vi "UHR-Fleezers Control (host) -Leonardo 04-2018 V3.vi"(0 "Tab Control":T5(tab)=enum."Trap Control (RF)") -> ()   [LabVIEW 2013] (continued)
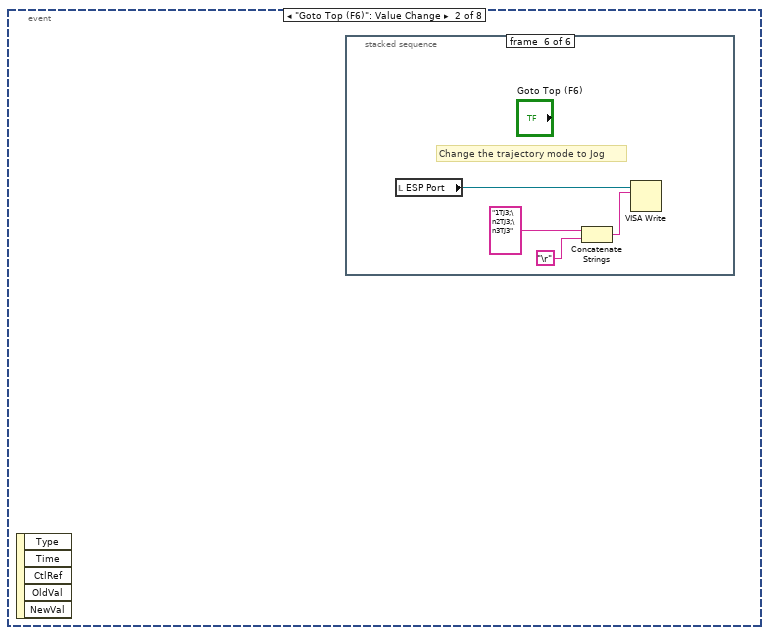
[diagram p4: hidden frame]
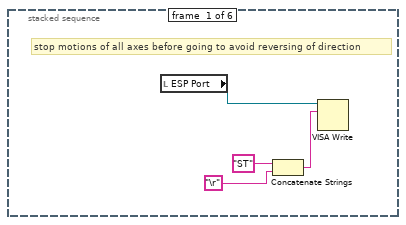
[diagram p5: hidden frame]
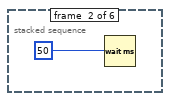
[diagram p6: hidden frame]
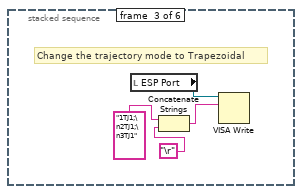
[diagram p7: hidden frame]
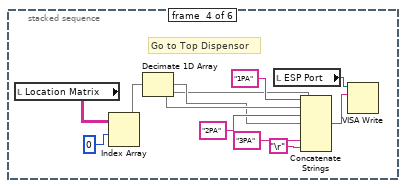
[diagram p8: hidden frame]
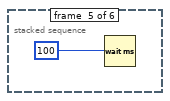
[diagram p9: hidden frame]
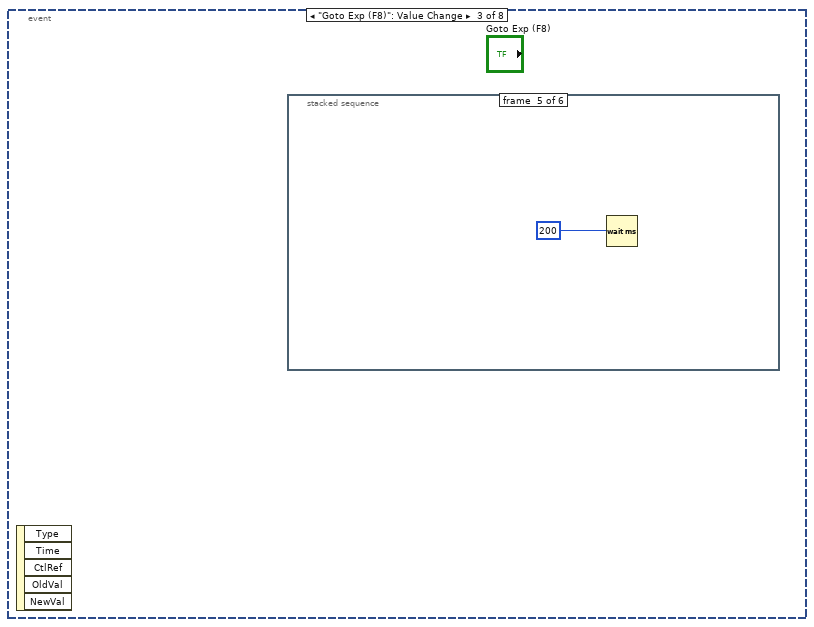
[diagram p10: hidden frame]
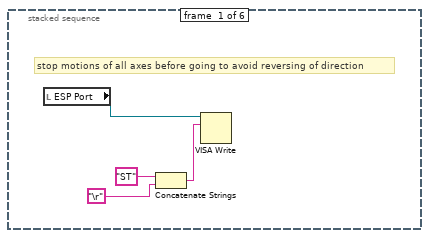
[diagram p11: hidden frame]
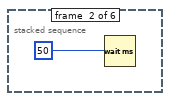
[diagram p12: hidden frame]
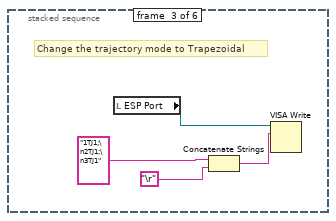
[diagram p13: hidden frame]
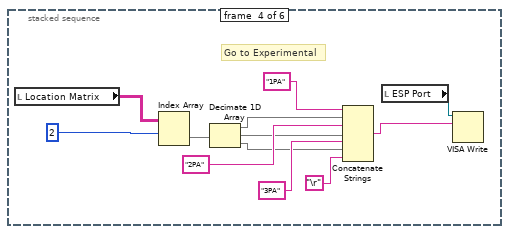
[diagram p14: hidden frame]
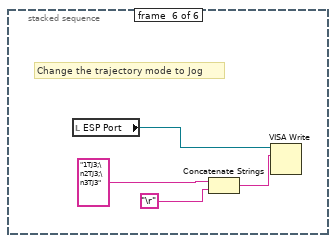
[diagram p15: hidden frame]
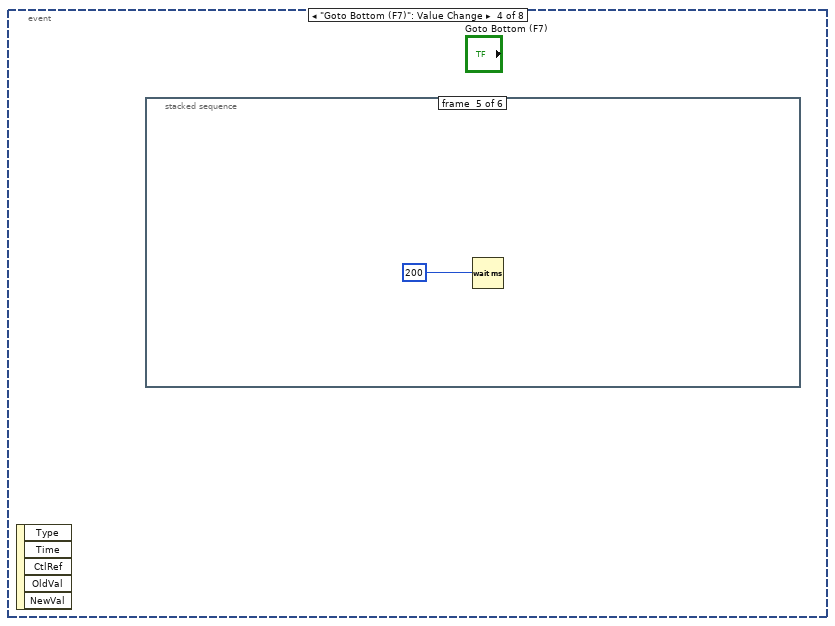
[diagram p16: hidden frame]
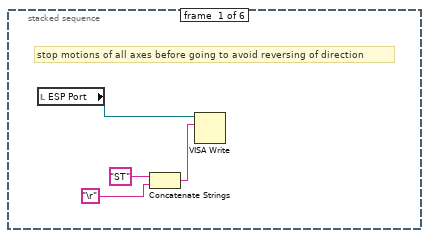
[diagram p17: hidden frame]
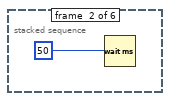
[diagram p18: hidden frame]
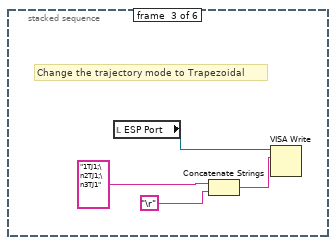
[diagram p19: hidden frame]
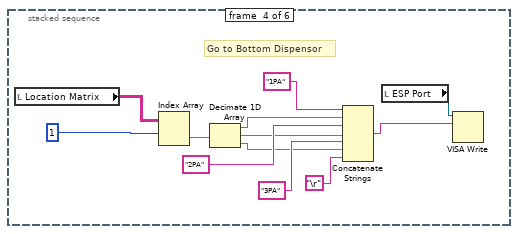
[diagram p20: hidden frame]
                n2319 = Write to Binary File(file (use dialog)=w3910, data=w3903, 5:FALSE ("prepend array or string size? (T)"), 9:T30."big-endian, network order" ("byte order (0:big-endian, network order)")) -> ()  [unwired: 1 in, 4 out]
                n2320 = feedback #26(w3876) -> (w3878:dbl[])
                n2321 = Build Array (concatenate)(w3878, w3876) -> (w3877:dbl[])
                n2322 = Select(t=w3876, s=w3852, f=w3877) -> (s? t:f=w3862:dbl[])
                n2323 = feedback-in #26(w3862) -> ()
                n2324 = feedback #27(w3884) -> (w3897:dbl[])
                n2325 = Build Array (concatenate)(w3897, w3884) -> (w3896:dbl[])
                n2326 = Select(t=w3884, s=w3852, f=w3896) -> (s? t:f=w3871:dbl[])
                n2327 = feedback-in #27(w3871) -> ()
                n2328 = Divide(x=w3911, y=w3912) -> (x/y=w3914:dbl)
                n2329 = Multiply(x=w3914, y=100.0) -> (x*y=w3913:dbl)
                n2330 = Build Array(w3871, w3862) -> (→"Saved APD":dbl[][])
                n2331 = Array Size(array=w3871) -> (size(s)=w3889:i32)
                n2332 = Unbundle By Name(w3891) -> ("Y"=w3895:dbl[])
                n2333 = Subtract(x=w3889, y="N pts to average") -> (x-y=w3865:i32)
                n2334 = Multiply(x="N pts to average", y=u16 2) -> (x*y=w3866:u16)
                n2335 = Subtract(x=w3889, y=w3866) -> (x-y=w3864:i32)
                n2336 = feedback #28(w3895) -> (w3894:dbl[])
                n2337 = Build Array (concatenate)(w3894, w3895) -> (w3893:dbl[])
                n2338 = Select(t=w3895, s=w3852, f=w3893) -> (s? t:f=w3892:dbl[])
                "Trap Delta Graph" <- w3892
                n2339 = feedback-in #28(w3892) -> ()
                n2340 = Array Subset(array=w3871, index=w3865, length="N pts to average") -> (w3888:dbl[])
                n2341 = Array Subset(array=w3871, index=w3864, length="N pts to average") -> (w3887:dbl[])
                n2342 = Array Subset(array=w3862, index=w3865, length="N pts to average") -> (w3868:dbl[])
                n2343 = Array Subset(array=w3862, index=w3864, length="N pts to average") -> (w3867:dbl[])
                n2344 = call-poly <vilib>:"Mean.vi"("X"=w3888) -> ("mean"=w3886:dbl)  [unwired: 1 out]
                n2345 = call-poly <vilib>:"Mean.vi"("X"=w3868) -> ("mean"=w3861:dbl)  [unwired: 1 out]
                n2346 = call-poly <vilib>:"Mean.vi"("X"=w3887) -> ("mean"=w3885:dbl)  [unwired: 1 out]
                n2347 = call-poly <vilib>:"Mean.vi"("X"=w3867) -> ("mean"=w3860:dbl)  [unwired: 1 out]
                n2348 = Subtract(x=w3861, y=w3860) -> (x-y=w3851:dbl)
                "Delta Fl. 2" <- w3851
                n2349 = Subtract(x=w3886, y=w3885) -> (x-y=w3883:dbl)
                "Delta Fl. 1" <- w3883
                n2350 = Initialize Array(w3883, 1 ("dimension size")) -> (w3880:dbl[])
                n2351 = Initialize Array(w3851, 1 ("dimension size")) -> (w3857:dbl[])
                n2352 = feedback #29(w3880) -> (w3881:dbl[])
                n2353 = Build Array (concatenate)(w3881, w3880) -> (w3879:dbl[])
                n2354 = feedback #30(w3857) -> (w3858:dbl[])
                n2355 = Build Array (concatenate)(w3858, w3857) -> (w3856:dbl[])
                n2356 = Select(t=w3880, s=w3852, f=w3879) -> (s? t:f=w3855:dbl[])
                n2357 = feedback-in #29(w3855) -> ()
                n2358 = Select(t=w3857, s=w3852, f=w3856) -> (s? t:f=w3854:dbl[])
                n2359 = feedback-in #30(w3854) -> ()
                n2360 = Build Array(w3855, w3854) -> (→"Save APD Deriv":dbl[][])
              }
            }
            "Progress" <- w3828
            "Progress 2" <- w3828
          }
        }
      }
    }
    n2361 = Divide(x=w2209, y=w2210) -> (x/y=w2200:ext)
    "Trap 2 amplitude" <- w2200
    n2362 = Bundle By Name(cluster=w2463, "Green FB Ch 0"=w2462, "Green FB Ch 1"=w2461) -> (w2447:T49)
    "Green FB Signals (V)" <- w2447
    n2363 = case shown="True" w2202 {
      tunnel: w2201 -> [_ w2552]
      tunnel: w2200 -> [_ w2551]
      frame False {
      }
      frame True {
        w2553 = 50.0
        n2364 = Greater?(x=w2551, y=w2553) -> (0:w2549:bool)
        n2365 = Greater?(x=w2552, y=w2553) -> (0:w2550:bool)
        n2366 = Or(x=w2550, y=w2549) -> (x .or. y?=w2548:bool)
        n2367 = case shown="True" w2548 {
          frame False {
          }
          frame True {
            n2368 = property on="All FB On/Off" class="Bool (strict)"("Val(Sgnl)"=FALSE) -> ()  [unwired: 2 in, 2 out]
            "Feedback overload" <- TRUE
          }
        }
      }
    }
    n2369 = Unbundle By Name(w2447) -> ("Green FB Ch 2"=→"Green FB Plot":dbl)
    n2370 = local read "wait to reset values"() -> (w2531:bool)
    n2371 = Not(x=w2528) -> (.not. x?=w2532:bool)
    n2372 = And(x=w2532, y=w2531) -> (x .and. y?=w2533:bool)
    n2373 = case "Part of MCL raster scanning: returns to initial positions after scan done" shown="True" w2533 {
      tunnel: w2536 -> [w3377 w3384]
      tunnel: [w3377 w3383] -> w2535
      tunnel: w2530 -> [w3376 w3382]
      tunnel: [w3376 w3381] -> w2529
      frame False {
      }
      frame True {
        w3392 = 10.0 ("y")
        w3391 = 32767.0 ("y")
        # "to return scan values\nafter a synchronous \nAOM scan"
        n2374 = local read "AO2"() -> (w3385:dbl)
        n2375 = local read "AO1"() -> (w3386:dbl)
        n2376 = local write "wait to reset values"(FALSE ("wait to reset values")) -> ()
        n2377 = Multiply(x=w3386, y=w3391) -> (x*y=w3388:dbl)
        n2378 = Multiply(x=w3385, y=w3391) -> (x*y=w3390:dbl)
        n2379 = Divide(x=w3388, y=w3392) -> (x/y=w3387:dbl)
        n2380 = Divide(x=w3390, y=w3392) -> (x/y=w3389:dbl)
        n2381 = To Word Integer(number=w3387) -> (16bit integer=w3393:i16)
        n2382 = To Word Integer(number=w3389) -> (16bit integer=w3394:i16)
        n2383 = local read "Total Counts (ticks)"() -> (w3378:u32)
        n2384 = xnode "Read/Write Control"("FPGA VI Reference In"=w3384, "error in"=w3382, "AO1 (Y)"=w3393, "AO2 (X)"=w3394, "MCL count"=w3378) -> ("FPGA VI Reference Out"=w3383:T20, "error out"=w3381:errorcluster)
        n2385 = local read "Scan Range (V)\n(of steps)"() -> (w3379:dbl)
        n2386 = property on="Scan Range (V)\n(of steps)" class="DigNum (strict)"("Val(Sgnl)"=w3379) -> ()  [unwired: 2 in, 2 out]
      }
    }
    n2387 = node-c288() -> ()  [unwired: 2 out]
  }
  n2388 = node-c288(3 ("Processor")) -> (w107:T25)  [unwired: 3 out]
  n2389 = timed-loop "Oscillate AOD (debugging)" {
    tunnel: w57 -> [w3956]
    tunnel: [w3955] -> w69
    timing: w107 -> [_]
    timing-out: [_] -> w106
    stop <- w3955 stop-if-true
    n2390 = node-c288() -> ()  [unwired: 2 out]
    n2391 = event shown="[0] \"Oscillate Set 2\", \"Fish for Tether\": Value Change" {
      selector: _ -> [_ _ _]
      dyn-events: _ -> [_ _ _]
      timeout: _ -> [_ _ _]
      tunnel: w3956 -> [w3963 _ _]
      tunnel: [FALSE ("Stop All") _ w4231] -> w3955
      event "Oscillate Set 2", "Fish for Tether": Value Change {
        n2392 = event-data() -> ()  [unwired: 6 out]
        n2393 = local read "Oscillate Set 2"() -> (w3962:bool)
        n2394 = Or(x=w3962, y="Fish for Tether") -> (x .or. y?=w3960:bool)
        n2395 = case shown="True" w3960 {
          tunnel: w3963 -> [_ w3966]
          tunnel: "Fish for Tether" -> [_ w3965]
          frame False {
          }
          frame True {
            n2396 = case shown="True" w3965 {
              frame False {
              }
              frame True {
                n2397 = local write "Scan axis 2"(TRUE) -> ()
                n2398 = local write "Tether"(FALSE ("Tether")) -> ()
              }
            }
            n2399 = node-c288("Period") -> (w3968:T25)  [unwired: 3 out]
            n2400 = timed-loop "Oscillate AOD" {
              timing: w3968 -> [_]
              timing-out: [_] -> w3967
              tunnel: w3966 -> [w3978]
              tunnel: w3965 -> [w3977]
              i -> [w3980]
              stop <- w3976 stop-if-true
              n2401 = node-c288() -> (w3979:i64)  [unwired: 1 out]
              n2402 = flat-sequence {
                tunnel: w3980 -> [w4006]
                tunnel: w3979 -> [w4005]
                tunnel: w3978 -> [w3989]
                tunnel: w3977 -> [w3991]
                tunnel: [w3991] -> w3975
                tunnel: [w3990] -> w3974
                tunnel: [w3988] -> w3973
                tunnel: [w3985] -> w3971
                tunnel: w3975 -> [w4042]
                tunnel: w3974 -> [w4040]
                tunnel: w3973 -> [w4039]
                tunnel: [w4038] -> w3972
                tunnel: w3971 -> [w4037]
                tunnel: [w4106] -> w3976
                tunnel: w3972 -> [w4104]
                frame #0 {
                  n2403 = Divide(x=w4005, y=i64 1000) -> (x/y=w4000:dbl)
                  n2404 = Multiply(x=w4000, y=w4006) -> (x*y=w4002:dbl)
                  n2405 = Multiply(x="Osc. freq. (Hz)", y=6.283185307179586) -> (x*y=w4003:dbl)
                  n2406 = Multiply(x=w4003, y=w4002) -> (x*y=w3987:dbl)
                  n2407 = local read "BD 1 Frequency 2 (MHz)"() -> (w3984:dbl)
                  n2408 = local read "BD 1 Frequency 1 (MHz)"() -> (w3981:dbl)
                  n2409 = case shown="True" w3991 {
                    tunnel: w3987 -> [w4012 w4019]
                    tunnel: w3984 -> [_ w4029]
                    tunnel: [w4009 w4013] -> w3992
                    tunnel: [FALSE w4022] -> w3988
                    tunnel: [0.0 w4015] -> w3985
                    tunnel: w3981 -> [_ w4014]
                    frame False {
                      n2410 = Sine(x=w4012) -> (sin(x)=w4010:dbl)
                      n2411 = Multiply(x=w4010, y="Osc. amp. (MHz)") -> (x*y=w4009:dbl)
                    }
                    frame True {
                      n2412 = Cosine(x=w4019) -> (cos(x)=w4032:dbl)
                      n2413 = Subtract(x=w4029, y=w4014) -> (x-y=w4028:dbl)
                      n2414 = Decrement(x=w4032) -> (x-1=w4031:dbl)
                      n2415 = Subtract(x=w4028, y="Closest Delta (MHz)") -> (x-y=w4025:dbl)
                      n2416 = Divide(x=w4031, y=2.0) -> (x/y=w4026:dbl)
                      n2417 = Multiply(x=w4026, y=w4025) -> (x*y=w4013:dbl)
                      n2418 = local read "Vec Mean of T1 T2"() -> (w4021:dbl[])
                      n2419 = Greater?(x=w4021, y="Stop F (pN)") -> (0:w4023:bool[])
                      n2420 = Or Array Elements(Boolean array=w4023) -> (logical OR=w4022:bool)
                      n2421 = Divide(x=w4019, y=6.283185307179586) -> (x/y=w4018:dbl)
                      n2422 = Round Toward +Infinity(x=w4018) -> (ceil(x): smallest int >= x=w4015:dbl)
                      "Attempts" <- w4015
                      n2423 = Greater?(x=w4015, y="Attempt Limit") -> (0:w4017:bool)
                      n2424 = case shown="True" w4017 {
                        frame False {
                        }
                        frame True {
                          n2425 = local write "Fish for Tether"(FALSE ("Fish for Tether")) -> ()
                          n2426 = call <vilib>:"Beep.vi"() -> ()  [unwired: 3 in, 9 out]
                          n2427 = local read "Messages"() -> (w4034:string)
                          n2428 = call "Update messages.vi"("Message to add"="Tether fishing timeout." ("Messages"), "Old message string"=w4034) -> ("New message string"=→"Messages":string)
                        }
                      }
                    }
                  }
                  n2429 = local read "Y RF Frequency Limits (MHz)"() -> (w3993:T16)
                  n2430 = local read "X RF Frequency Limits (MHz)"() -> (w3994:T16)
                  n2431 = local read "BD 1 Frequency 3 (MHz)"() -> (w3999:dbl)
                  n2432 = local read "BD 2 Frequency 2 (MHz)"() -> (w3983:dbl)
                  n2433 = Select(t=w3984, s="Scan axis 2", f=w3983) -> (s? t:f=w3995:dbl)
                  n2434 = Add(x=w3992, y=w3995) -> (x+y=w3990:dbl)
                  n2435 = Select(t=w3990, s="Scan axis 2", f=w3984) -> (s? t:f=w3982:dbl)
                  n2436 = Select(t=w3983, s="Scan axis 2", f=w3990) -> (s? t:f=w3997:dbl)
                  n2437 = local read "BD 2 Frequency 3 (MHz)"() -> (w3998:dbl)
                  n2438 = call "set RF board frequency - interlace.vi"("Board 2 Frequency Limits"=w3993, "Board 1 Frequency Limits"=w3994, "FPGA VI Reference In"=w3989, "Board 2 Frequency 3 (MHz)"=w3998, "Board 1 Frequency 3 (MHz)"=w3999, "Board 2 Frequency 2 (MHz)"=w3983, "Board 2 Frequency 1 (MHz)"=w3997, "Board 1 Frequency 2 (MHz)"=w3982, "Board 1 Frequency 1  (MHz)"=w3981) -> ()  [unwired: 1 in, 2 out]
                }
                frame #1 {
                  n2439 = And(x=w4042, y=w4039) -> (x .and. y?=w4041:bool)
                  n2440 = case "Only if were fishing and now formed tether" shown="True" w4041 {
                    tunnel: w4040 -> [w4044 w4056]
                    tunnel: [w4043 w4055] -> w4038
                    tunnel: w4037 -> [_ w4051]
                    frame False {
                      n2441 = local read "Fish for Tether"() -> (w4043:bool)
                      n2442 = case shown="True" w4043 {
                        tunnel: w4044 -> [_ _]
                        frame False {
                        }
                        frame True {
                        }
                      }
                    }
                    frame True {
                      w4055 = FALSE ("Fish for Tether")
                      n2443 = call <vilib>:"Beep.vi"() -> ()  [unwired: 3 in, 9 out]
                      n2444 = Number To Decimal String(number=w4051, width (-)=i16 1) -> (decimal integer string=w4049:string)
                      n2445 = case shown="\"2\", \"3\", \"4\", \"5\", \"6\"" "Then..." {
                        selector: "Then..." -> [_ w4059]
                        tunnel: w4056 -> [w4058 _]
                        frame "1", Default {
                          # "do nothing"
                          n2446 = property on="BD 1 Frequency 1 (MHz)" class="DigNum (strict)"("Val(Sgnl)"=w4058) -> ()  [unwired: 2 in, 2 out]
                        }
                        frame "2", "3", "4", "5", "6" {
                          n2447 = flat-sequence {
                            tunnel: w4059 -> [w4061]
                            frame #0 {
                              n2448 = property on="Trap Delta (MHz)" class="DigNum (strict)"("Val(Sgnl)"="Move to Delta 1 (MHz)") -> ()  [unwired: 2 in, 2 out]
                            }
                            frame #1 {
                              n2449 = case shown="\"5\", \"6\"" w4061 {
                                selector: w4061 -> [w4064 w4074 _]
                                frame "3", "4" {
                                n2450 = flat-sequence {
                                tunnel: w4064 -> [w4065]
                                tunnel: [w4065] -> w4062
                                tunnel: [w4067] -> w4063
                                tunnel: w4062 -> [w4067]
                                tunnel: w4063 -> [w4071]
                                frame #0 {
                                n2451 = property on="Green Laser ON/Interlacing" class="Bool (strict)"("Val(Sgnl)"=TRUE ("Value (Signaling)")) -> ()  [unwired: 2 in, 2 out]
                                }
                                frame #1 {
                                n2452 = Multiply(x="Wait Before Save (s)", y=u32 1000 ("x")) -> (x*y=w4069:u32)
                                n2453 = Wait (ms)(milliseconds to wait=w4069) -> ()  [unwired: 1 out]
                                }
                                frame #2 {
                                n2454 = property on="Start Saving" class="Bool (strict)"("Value"=TRUE ("Start Saving")) -> ()  [unwired: 2 in, 2 out]
                                n2455 = case shown="Default" w4071 {
                                frame Default {
                                }
                                frame "4" {
                                n2456 = property on="Fl. Triggered..." class="Bool (strict)"("Val(Sgnl)"=TRUE ("Value (Signaling)")) -> ()  [unwired: 2 in, 2 out]
                                }
                                }
                                }
                                }
                                }
                                frame "5", "6" {
                                n2457 = stacked-sequence {
                                tunnel: w4074 -> [_ _ _ _ _ _ _ _ w4091 _ _]
                                frame #0 {
                                n2458 = Replace Array Subset(array=u32[] [0] ("Index Values"), new element="Raster Set Upon Tether", index=0) -> (w4075:u32[])
                                n2459 = property on="Saved AOD Raster Scan Parameter Sets" class="Arr (strict)"("Index Values"=w4075) -> ()  [unwired: 2 in, 2 out]
                                }
                                frame #1 {
                                n2460 = Wait (ms)(milliseconds to wait=u32 500) -> ()  [unwired: 1 out]
                                }
                                frame #2 {
                                n2461 = property on="Load parameters" class="Bool (strict)"("Val(Sgnl)"=TRUE ("Value (Signaling)")) -> ()  [unwired: 2 in, 2 out]
                                }
                                frame #3 {
                                n2462 = Wait (ms)(milliseconds to wait=u32 500) -> ()  [unwired: 1 out]
                                }
                                frame #4 {
                                n2463 = property on="Trap Raster Scan" class="Bool (strict)"("Val(Sgnl)"=TRUE ("Value (Signaling)")) -> ()  [unwired: 2 in, 2 out]
                                }
                                frame #5 {
                                n2464 = Wait (ms)(milliseconds to wait=u32 2000) -> ()  [unwired: 1 out]
                                }
                                frame #6 {
                                n2465 = while {
                                stop <- w4086 stop-if-true
                                n2466 = local read "Raster Scanning..."() -> (w4085:bool)
                                n2467 = local read "Saving..."() -> (w4088:bool)
                                n2468 = Wait (ms)(milliseconds to wait=u32 100) -> ()  [unwired: 1 out]
                                n2469 = Not(x=w4088) -> (.not. x?=w4087:bool)
                                n2470 = Not(x=w4085) -> (.not. x?=w4084:bool)
                                n2471 = And(x=w4087, y=w4084) -> (x .and. y?=w4086:bool)
                                }
                                }
                                frame #7 {
                                n2472 = property on="Trap Delta (MHz)" class="DigNum (strict)"("Val(Sgnl)"="Move to Delta 2 (MHz)") -> ()  [unwired: 2 in, 2 out]
                                }
                                frame #8 {
                                n2473 = local read "Tether"() -> (w4092:bool)
                                n2474 = case shown="True" w4092 {
                                tunnel: w4091 -> [_ w4093]
                                frame False {
                                }
                                frame True {
                                n2475 = flat-sequence {
                                tunnel: w4093 -> [w4095]
                                frame #0 {
                                n2476 = Wait (ms)(milliseconds to wait=u32 500) -> ()  [unwired: 1 out]
                                }
                                frame #1 {
                                n2477 = case shown="\"6\"" w4095 {
                                frame Default {
                                }
                                frame "6" {
                                n2478 = property on="Green Laser ON/Interlacing" class="Bool (strict)"("Val(Sgnl)"=TRUE ("Green Laser ON/Interlacing")) -> ()  [unwired: 2 in, 2 out]
                                }
                                }
                                }
                                frame #2 {
                                n2479 = Wait (ms)(milliseconds to wait=u32 500) -> ()  [unwired: 1 out]
                                }
                                frame #3 {
                                n2480 = local write "Start Saving"("Save at end (5, 6)") -> ()
                                }
                                }
                                }
                                }
                                }
                                frame #9 {
                                n2481 = local read "Bead Sep. Int. Time (s)"() -> (w4101:dbl)
                                n2482 = Multiply(x=w4101, y=1000.0) -> (x*y=w4100:dbl)
                                n2483 = Wait (ms)(milliseconds to wait=w4100) -> ()  [unwired: 1 out]
                                }
                                frame #10 {
                                n2484 = property on="Rescale on Mean" class="Bool (strict)"("Val(Sgnl)"=TRUE ("Value (Signaling)")) -> ()  [unwired: 2 in, 2 out]
                                }
                                }
                                }
                                frame "2", Default {
                                }
                              }
                            }
                          }
                        }
                      }
                      n2485 = Concatenate Strings("Formed tether in ", w4049, " attempt(s)." ("string")) -> (w4046:string)
                      n2486 = local read "Messages"() -> (w4053:string)
                      n2487 = local write "Fish for Tether"(w4055) -> ()
                      n2488 = call "Update messages.vi"("Message to add"=w4046, "Old message string"=w4053) -> ("New message string"=w4052:string)
                      n2489 = local write "Messages"(w4052) -> ()
                      n2490 = Get Date/Time In Seconds() -> (seconds since 1Jan1904=→"Time tether formed":timestamp)
                      "Tether" <- "Tether Alarm?"
                    }
                  }
                }
                frame #2 {
                  n2491 = local read "Oscillate Set 2"() -> (w4105:bool)
                  n2492 = local read "Stop All"() -> (w4107:bool)
                  n2493 = Not Or(1:w4104, 2:w4105) -> (0:w4103:bool)
                  n2494 = Compound Arithmetic op=OR(w4107, w4103) -> (w4106:bool)
                }
              }
              n2495 = node-c288() -> ()  [unwired: 2 out]
            }
            n2496 = node-c288(w3967) -> ()  [unwired: 1 out]
          }
        }
      }
      event "Fl. Triggered...": Value Change {
        n2497 = event-data() -> ()  [unwired: 7 out]
        n2498 = case shown="True" "Fl. Triggered..." {
          frame False {
          }
          frame True {
            n2499 = node-c288() -> (w4119:T25)  [unwired: 4 out]
            n2500 = timed-loop {
              timing: w4119 -> [_]
              timing-out: [_] -> w4118
              tunnel: "Action" -> [w4123]
              shift-right: [w4120] -> _
              shift-left: u8 255 -> [w4122]
              stop <- w4124 stop-if-true
              n2501 = node-c288() -> ()  [unwired: 2 out]
              n2502 = flat-sequence {
                tunnel: w4123 -> [w4136]
                tunnel: w4122 -> [w4133]
                tunnel: [w4132] -> w4121
                tunnel: [w4222] -> w4124
                tunnel: w4121 -> [w4221]
                tunnel: [w4221] -> w4120
                frame #0 {
                  n2503 = local read "Delta Fl. 2"() -> (w4127:dbl)
                  n2504 = local read "Delta Fl. 1"() -> (w4128:dbl)
                  n2505 = Select(t=w4128, s="APD to Watch", f=w4127) -> (s? t:f=w4126:dbl)
                  n2506 = Multiply(x="Fl. Delta Thresh. (kHz)", y=1000.0) -> (x*y=w4135:dbl)
                  n2507 = Greater?(x=w4126, y=w4135) -> (0:w4130:bool)
                  n2508 = Or(x="Force Yank", y=w4130) -> (x .or. y?=w4131:bool)
                  n2509 = case shown="True" w4131 {
                    tunnel: w4136 -> [_ w4146]
                    tunnel: w4133 -> [w4138 w4142]
                    tunnel: [w4138 w4139] -> w4132
                    frame False {
                    }
                    frame True {
                      n2510 = flat-sequence {
                        tunnel: w4143 -> [w4152]
                        tunnel: [w4152] -> w4147
                        tunnel: w4146 -> [w4151]
                        tunnel: [w4151] -> w4145
                        tunnel: [w4150] -> w4144
                        tunnel: w4142 -> [w4149]
                        tunnel: [w4148] -> w4141
                        tunnel: w4147 -> [w4177]
                        tunnel: w4145 -> [w4176]
                        tunnel: w4144 -> [w4175]
                        tunnel: w4141 -> [w4174]
                        tunnel: [w4174] -> w4140
                        tunnel: w4140 -> [w4219]
                        tunnel: [w4219] -> w4139
                        frame #0 {
                          n2511 = call <vilib>:"Beep.vi"() -> ()  [unwired: 3 in, 9 out]
                          n2512 = local write "Waiting"(FALSE ("Waiting")) -> ()
                          n2513 = Increment(x=w4149) -> (x+1=w4148:u8)
                          n2514 = case shown="\"Yank\"" w4151 {
                            tunnel: w4148 -> [_ _ w4158]
                            frame "Image" {
                              n2515 = property on="Confocal Image" class="Bool (strict)"("Val(Sgnl)"=TRUE ("Value (Signaling)")) -> ()  [unwired: 2 in, 2 out]
                            }
                            frame "Alarm", Default {
                            }
                            frame "Yank" {
                              n2516 = flat-sequence {
                                tunnel: w4158 -> [w4161]
                                tunnel: [w4160] -> w4157
                                tunnel: ["N Array El"] -> w4156
                                tunnel: w4157 -> [w4171]
                                tunnel: w4156 -> [w4167]
                                frame #0 {
                                n2517 = Multiply(x="Yank Delay (s)", y=1000.0) -> (x*y=w4164:dbl)
                                n2518 = Quotient & Remainder(x=w4161, y="N Array El") -> (x-y*floor(x/y)=w4160:u8)  [unwired: 1 out]
                                n2519 = Wait (ms)(milliseconds to wait=w4164) -> ()  [unwired: 1 out]
                                }
                                frame #1 {
                                n2520 = Random Number (0-1)() -> (number: 0 to 1=w4168:dbl)
                                n2521 = Multiply(x=w4167, y=w4168) -> (x*y=w4166:dbl)
                                n2522 = Round Toward -Infinity(1:w4166) -> (0:w4165:dbl)
                                n2523 = Select(t=w4165, s="Random Choice", f=w4171) -> (s? t:f=w4169:dbl)
                                n2524 = Index Array(array="Yank to Delta Array (MHz)", index=w4169) -> (element=w4172:dbl)
                                n2525 = property on="Trap Delta (MHz)" class="DigNum (strict)"("Val(Sgnl)"=w4172) -> ()  [unwired: 2 in, 2 out]
                                }
                              }
                            }
                          }
                          n2526 = local read "Time (s)"() -> (w4150:dbl)
                          "Fl. High" <- TRUE ("Yanking")
                        }
                        frame #1 {
                          n2527 = node-c288() -> (w4179:T25)  [unwired: 4 out]
                          n2528 = timed-loop {
                            timing: w4179 -> [_]
                            timing-out: [_] -> w4178
                            tunnel: w4177 -> [w4195]
                            tunnel: w4176 -> [w4193]
                            tunnel: w4175 -> [w4192]
                            stop <- w4194 stop-if-true
                            n2529 = node-c288() -> ()  [unwired: 2 out]
                            n2530 = local read "Fl. Delta Thresh. (kHz)"() -> (w4187:dbl)
                            n2531 = local read "Fl. Triggered..."() -> (w4196:bool)
                            n2532 = local read "Delta Fl. 1"() -> (w4183:dbl)
                            n2533 = local read "Delta Fl. 2"() -> (w4181:dbl)
                            n2534 = local read "Stop All"() -> (w4190:bool)
                            n2535 = local read "APD to Watch"() -> (w4182:bool)
                            n2536 = Select(t=w4183, s=w4182, f=w4181) -> (s? t:f=w4180:dbl)
                            n2537 = Not(x=w4196) -> (.not. x?=w4191:bool)
                            n2538 = Multiply(x=w4187, y=1000.0) -> (x*y=w4186:dbl)
                            n2539 = Negate(x=w4186) -> (-x=w4185:dbl)
                            n2540 = Less?(x=w4180, y=w4185) -> (x < y?=w4189:bool)
                            n2541 = Compound Arithmetic op=OR(w4189, w4190, w4191, "Force Reset") -> (w4194:bool)
                            n2542 = case shown="True" w4194 {
                              tunnel: w4195 -> [_ w4207]
                              tunnel: w4193 -> [_ w4206]
                              tunnel: w4192 -> [_ w4204]
                              frame False {
                              }
                              frame True {
                                n2543 = case shown="\"Yank\"" w4206 {
                                tunnel: w4207 -> [_ w4208]
                                frame "Image", Default {
                                }
                                frame "Yank" {
                                n2544 = flat-sequence {
                                tunnel: [w4213] -> w4209
                                tunnel: w4208 -> [w4213]
                                tunnel: w4209 -> [w4214]
                                frame #0 {
                                n2545 = local read "Yank Delay (s)"() -> (w4212:dbl)
                                n2546 = Multiply(x=w4212, y=1000.0) -> (x*y=w4210:dbl)
                                n2547 = Wait (ms)(milliseconds to wait=w4210) -> ()  [unwired: 1 out]
                                }
                                frame #1 {
                                n2548 = property on="Trap Delta (MHz)" class="DigNum (strict)"("Val(Sgnl)"=w4214) -> ()  [unwired: 2 in, 2 out]
                                }
                                }
                                }
                                }
                                n2549 = local read "Time (s)"() -> (w4205:dbl)
                                n2550 = Subtract(x=w4205, y=w4204) -> (x-y=w4201:dbl)
                                "Duration (s)" <- w4201
                                n2551 = Number To Decimal String(number=w4201, width (-)=i16 0) -> (decimal integer string=w4199:string)
                                n2552 = Concatenate Strings(w4199, " s fluorescence event." ("string")) -> (w4197:string)
                                n2553 = local read "Messages"() -> (w4203:string)
                                n2554 = call "Update messages.vi"("Message to add"=w4197, "Old message string"=w4203) -> ("New message string"=w4202:string)
                                n2555 = call <vilib>:"Beep.vi"() -> ()  [unwired: 3 in, 9 out]
                                n2556 = local write "Messages"(w4202) -> ()
                              }
                            }
                            n2557 = node-c288() -> ()  [unwired: 2 out]
                          }
                          n2558 = node-c288(w4178) -> ()  [unwired: 1 out]
                        }
                        frame #2 {
                          n2559 = local write "Fl. High"(FALSE ("Yanking")) -> ()
                        }
                      }
                      n2560 = local read "Trap Delta (MHz)"() -> (w4143:dbl)
                    }
                  }
                }
                frame #1 {
                  n2561 = local read "Stop All"() -> (w4225:bool)
                  n2562 = local read "Fl. Triggered..."() -> (w4223:bool)
                  n2563 = Not(x=w4223) -> (.not. x?=w4224:bool)
                  n2564 = Or(x=w4224, y=w4225) -> (x .or. y?=w4222:bool)
                  n2565 = Not(x=w4222) -> (.not. x?=→"Waiting":bool)
                }
              }
              n2566 = node-c288() -> ()  [unwired: 2 out]
            }
            n2567 = node-c288(w4118) -> ()  [unwired: 1 out]
          }
        }
      }
      event "Stop All": Value Change {
        n2568 = event-data() -> ()  [unwired: 7 out]
        n2569 = local read "Stop All"() -> (w4231:bool)
      }
    }
    n2570 = node-c288() -> ()  [unwired: 2 out]
  }
  n2571 = node-c288(w106) -> ()  [unwired: 1 out]
  n2572 = node-c288(w193) -> ()  [unwired: 1 out]
  n2573 = flat-sequence {
    tunnel: w66 -> [w4236]
    tunnel: [w4235] -> w72
    tunnel: [w4232] -> w71
    tunnel: w70 -> [_]
    tunnel: w69 -> [_]
    tunnel: w68 -> [_]
    tunnel: w67 -> [_]
    tunnel: w65 -> [w4233]
    tunnel: w72 -> [w4239]
    tunnel: w71 -> [w4238]
    frame #0 {
      w4234 = FALSE ("APD to FIFO")
      n2574 = xnode "Read/Write Control"("FPGA VI Reference In"=w4236, "error in"=w4233, "APD to FIFO"=w4234, "AI to FIFO"=w4234) -> ("FPGA VI Reference Out"=w4235:T20, "error out"=w4232:errorcluster)
    }
    frame #1 {
      n2575 = xnode "Invoke Method"("FPGA VI Reference In"=w4239, "error in"=w4238) -> ("FPGA VI Reference Out"=w4237:T20)  [unwired: 1 out]
      n2576 = xnode "Close FPGA VI Reference"("FPGA VI Reference In"=w4237) -> ()  [unwired: 1 in, 1 out]
    }
  }
